vi "Clear Columns.vi"(11 "error in (no error)":errorcluster) -> (15 "error out":errorcluster)   [LabVIEW 2023, in "RFCalAndFixtureCharact.Common.lvlib"]
uses:
  RFCalAndFixtureCharact.Common.lvlib
  Type Definitions/Dictionary Operation.ctl
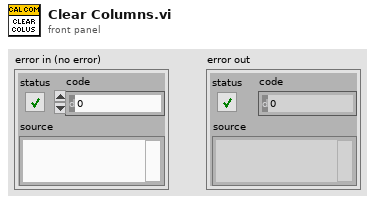
[diagram p1: front panel]
types:
  T1 = typedef "RFCalAndFixtureCharact.Common.lvlib/Dictionary Operation.ctl" = enum16{"Read", "Insert", "Remove", "Clear", "Get All", "Update"}
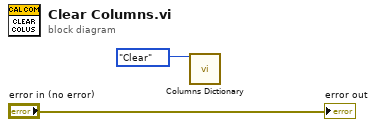
[diagram p0: block diagram]
diagram:
  n1 = call "Columns Dictionary.vi"("Action"=Dictionary_Operation."Clear") -> ()  [unwired: 12 in, 3 out]
  "error out" <- "error in (no error)"
